vi "tcp_senddata.vi"(8 "error In":errorcluster, 10 "array":dbl[](array[numeric]), 11 "Data In":T1) -> (0 "Error Out":errorcluster, 2 "# of Connections":i32, 3 "Data Out":T1)   [LabVIEW 2018]
panel:
  out "concatenated string":string
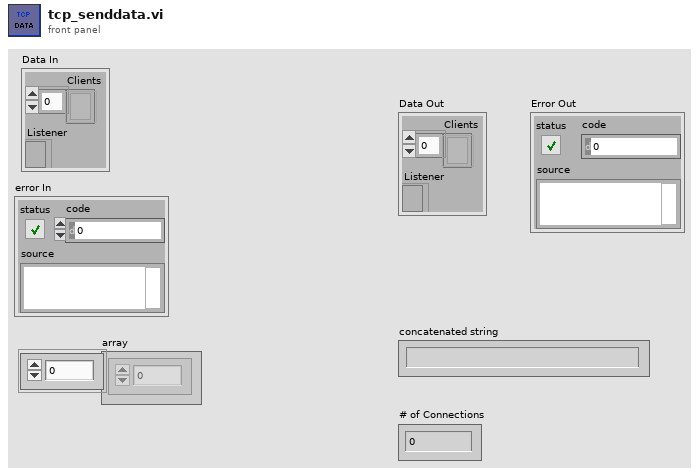
[diagram p1: front panel]
types:
  T1 = cluster{"Clients":refnum<k5>[], "Listener":refnum<k5>}
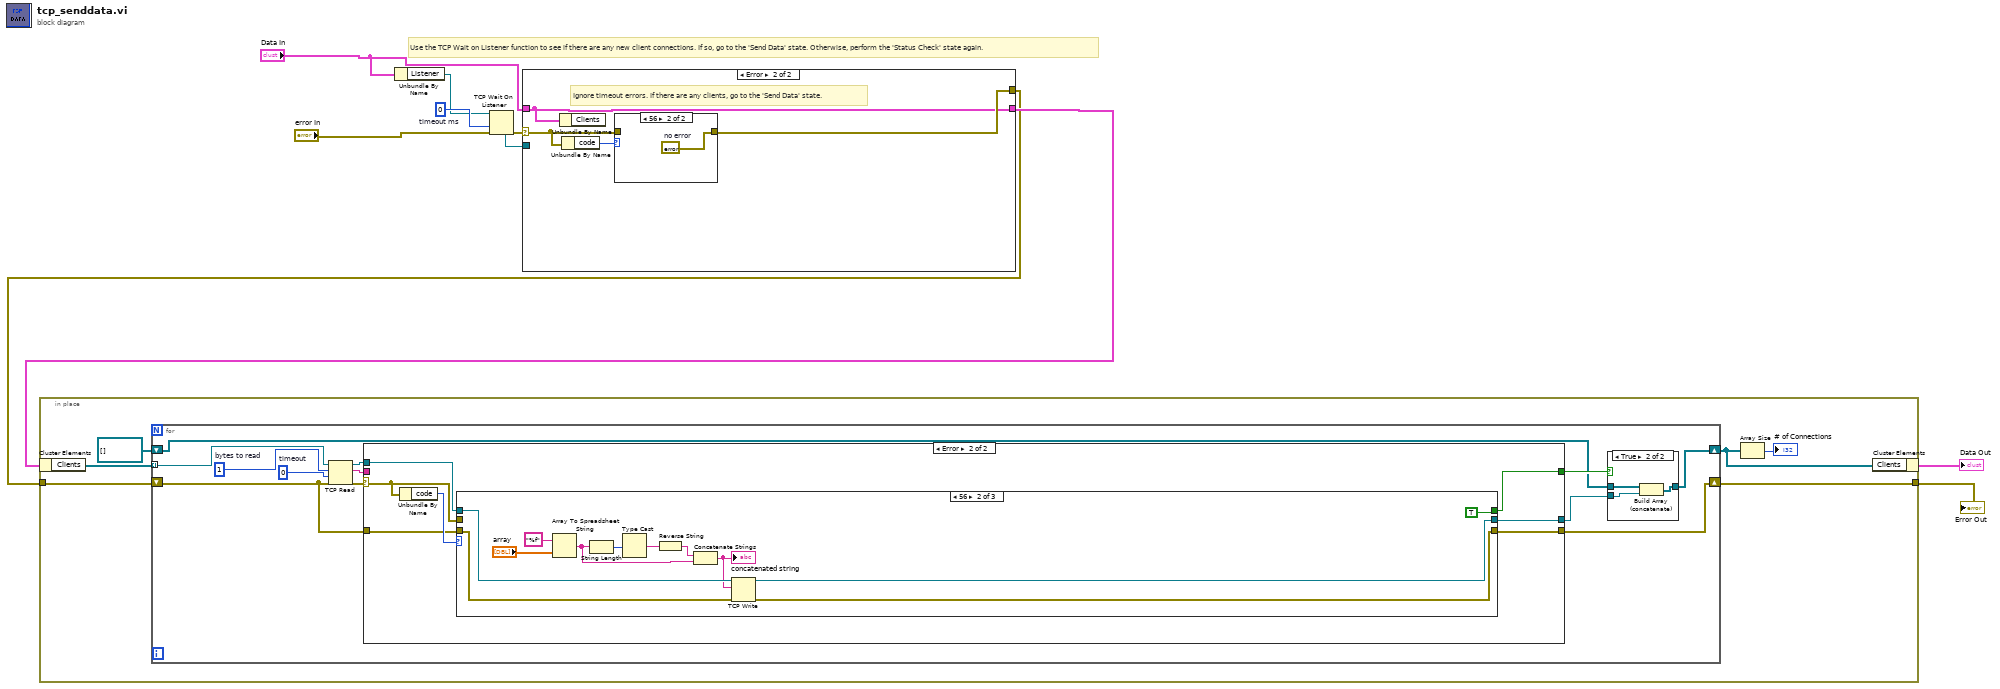
[diagram p0: block diagram]
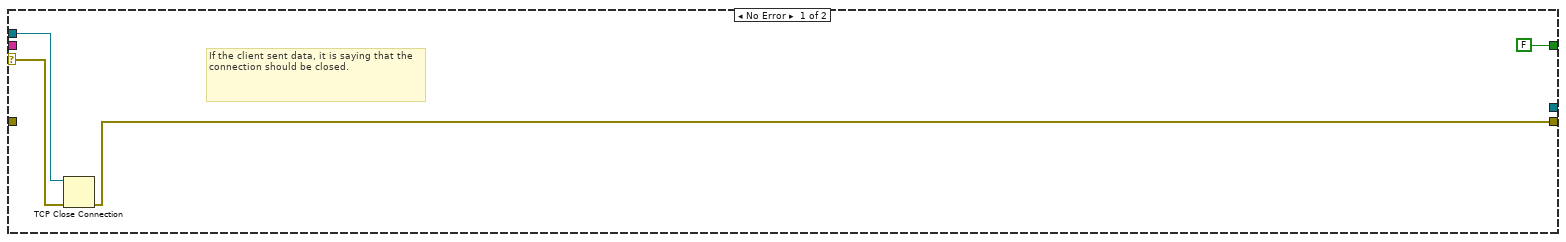
[diagram p3: hidden frame]
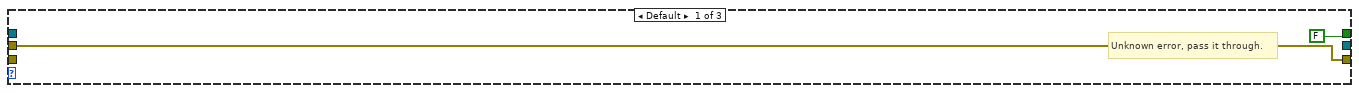
[diagram p4: hidden frame]
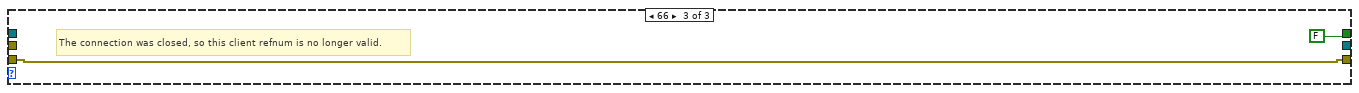
[diagram p5: hidden frame]
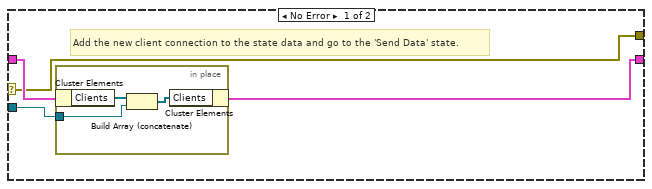
[diagram p6: hidden frame]
diagram:
  w10 = 0  # timeout ms
  # "Use the TCP Wait on Listener function to see if there are any new client connections. If so, go to the 'Send Data' state. Otherwise, perform the 'Status Check' state again."
  n1 = Unbundle By Name("Data In") -> ("Listener"=w7:refnum<k5>)
  n2 = TCP Wait On Listener(8:"error In", 9:w10, 11:w7) -> (0:w9:errorcluster, 4:w8:refnum<k5>)  [unwired: 4 out]
  n3 = case shown="Error" w9 {
    selector: w9 -> [w12 w21]
    tunnel: w8 -> [w13 _]
    tunnel: "Data In" -> [w14 w18]
    tunnel: [w11 w18] -> w5
    tunnel: [w12 w19] -> w4
    frame No Error {
      # "Add the new client connection to the state data and go to the 'Send Data' state."
      n4 = in-place {
        in-place-border: w13 -> [w15]
        n5 = in-place-cluster #1(w14) -> ("Clients"=w17:refnum<k5>[])
        n6 = Build Array (concatenate)(w17, w15) -> (w16:refnum<k5>[])
        n7 = in-place-cluster #1("Clients"=w16) -> (w11:T1)
      }
    }
    frame Error {
      # "Ignore timeout errors. If there are any clients, go to the 'Send Data' state."
      n8 = Unbundle By Name(w18) -> ()  [unwired: 1 out]
      n9 = Unbundle By Name(w21) -> ("code"=w20:i32)
      n10 = case shown="56" w20 {
        tunnel: w21 -> [w22 _]
        tunnel: [w22 w23] -> w19
        frame Default {
        }
        frame 56 {
          w23 = errorcluster {"status"=FALSE, "code"=0, "source"=""}  # no error
        }
      }
    }
  }
  n11 = in-place {
    in-place-border: w4 -> [w29]
    in-place-border: [w28] -> w2
    n12 = in-place-cluster #2(w5) -> ("Clients"=w26:refnum<k5>[])
    n13 = for {
      tunnel: w26 -> [w41] mode=indexing
      shift-right: [w33] -> w28
      shift-left: w29 -> [w32]
      shift-right: [w30] -> w25
      shift-left: refnum<k5>[] [] ("Array") -> [w31]
      w38 = 0  # timeout
      w39 = 1  # bytes to read
      n14 = TCP Read(connection ID=w41, bytes to read=w39, error in (no error)=w32, 9:w38) -> (connection ID out=w40:refnum<k5>, data out=w36:string, error out=w37:errorcluster)  [unwired: 1 out]
      n15 = case shown="Error" w37 {
        selector: w37 -> [w48 w55]
        tunnel: w40 -> [w49 w52]
        tunnel: w36 -> [_ _]
        tunnel: [_ w50] -> w35
        tunnel: [FALSE w51] -> w34
        tunnel: [w46 w54] -> w33
        tunnel: w32 -> [_ w53]
        frame No Error {
          # "If the client sent data, it is saying that the connection should be closed."
          # "If the client sent data, it is saying that the connection should be closed."
          n16 = TCP Close Connection(connection ID=w49, error in (no error)=w48) -> (error out=w46:errorcluster)  [unwired: 2 out]
        }
        frame Error {
          # "Ignore connection closed and timeout errors"
          n17 = Unbundle By Name(w55) -> ("code"=w56:i32)
          n18 = case shown="56" w56 {
            tunnel: w55 -> [w58 _ _]
            tunnel: [w58 w70 w72] -> w54
            tunnel: w53 -> [_ w66 w72]
            tunnel: w52 -> [_ w69 _]
            tunnel: [FALSE TRUE FALSE] -> w51
            tunnel: [_ w68 _] -> w50
            frame Default {
              # "Unknown error, pass it through."
            }
            frame 56 {
              n19 = Array To Spreadsheet String(array="array", 3:"%f" ("format string")) -> (spreadsheet string=w61:string)  [unwired: 1 in]
              n20 = String Length(string=w61) -> (length=w65:i32)
              n21 = Type Cast(x=w65) -> (*(type *) &x=w63:string)  [unwired: 1 in]
              n22 = Reverse String(1:w63) -> (0:w62:string)
              n23 = Concatenate Strings(w62, w61) -> (w64:string)
              "concatenated string" <- w64
              n24 = TCP Write(connection ID=w69, data in=w64, error in (no error)=w66) -> (connection ID out=w68:refnum<k5>, error out=w70:errorcluster)  [unwired: 2 out]
            }
            frame 66 {
              # "The connection was closed, so this client refnum is no longer valid."
            }
          }
        }
      }
      n25 = case shown="True" w34 {
        tunnel: w31 -> [w42 w44]
        tunnel: w35 -> [_ w43]
        tunnel: [w42 w45] -> w30
        frame False {
        }
        frame True {
          n26 = Build Array (concatenate)(w44, w43) -> (w45:refnum<k5>[])
        }
      }
    }
    n27 = Array Size(array=w25) -> (size(s)=→"# of Connections":i32)
    n28 = in-place-cluster #2("Clients"=w25) -> (→"Data Out":T1)
  }
  "Error Out" <- w2
